vi "GDFfindEventsOfSpecificType.vi"(10 "Selected Event Type":string, 11 "Array of Events in":T1[](array[typedef])) -> (2 "Number Of Events":i32, 3 "Array of Event Indexes":i32[](array[numeric]))   [LabVIEW 2016, in "GDF File Reader.lvlib"]
uses:
  GDF File Reader.lvlib
  EventDataType.ctl
panel:
  # "This VI is a part of BCI Design library, http://www.ru-bci.org \nCopyright © 2020, Sotnikov Peter, All rights reserved. License: CC BY-NC 4.0"
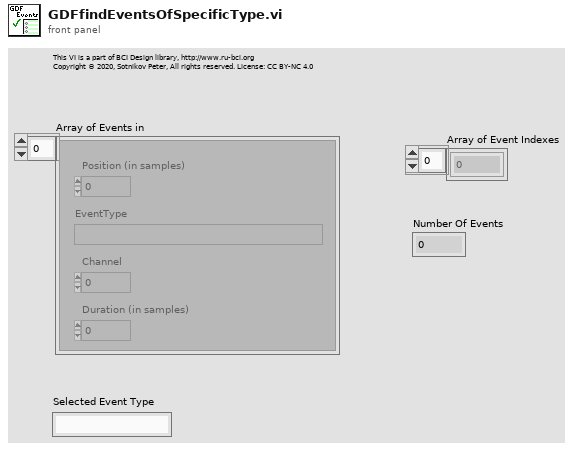
[diagram p1: front panel]
types:
  T1 = typedef "GDF File Reader.lvlib/EventDataType.ctl" = cluster{"Position (in samples)":u32, "EventType":string, "Channel":u16, "Duration (in samples)":u32}
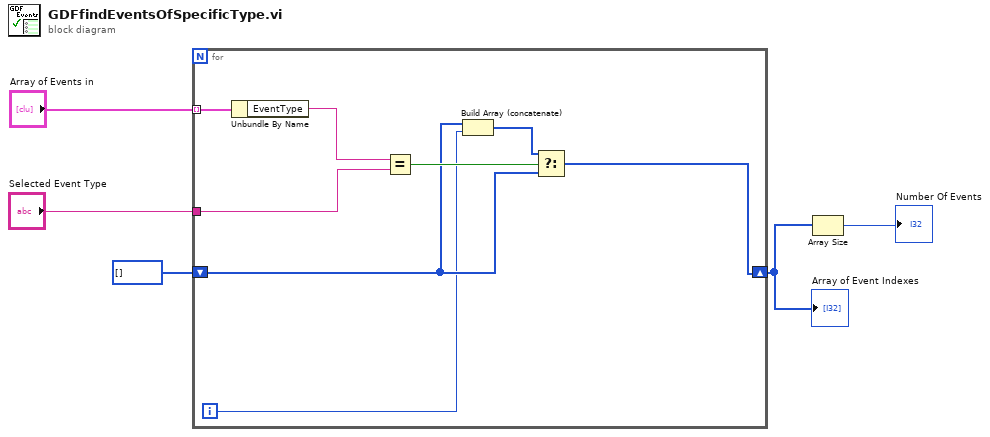
[diagram p0: block diagram]
diagram:
  n1 = for {
    tunnel: "Array of Events in" -> [w13] mode=indexing
    tunnel: "Selected Event Type" -> [w11]
    shift-right: [w6] -> w2
    shift-left: i32[] [] -> [w9]
    i -> [w8]
    n2 = Unbundle By Name(w13) -> ("EventType"=w12:string)
    n3 = Equal?(x=w12, y=w11) -> (x = y?=w10:bool)
    n4 = Build Array (concatenate)(w9, w8) -> (w7:i32[])
    n5 = Select(t=w7, s=w10, f=w9) -> (s? t:f=w6:i32[])
  }
  "Array of Event Indexes" <- w2
  n6 = Array Size(array=w2) -> (size(s)=→"Number Of Events":i32)
